vi "Experiment_1b.vi"() -> ()   [LabVIEW 2019]
uses:
  <vilib>/measure/NI_MABase.lvlib
panel:
  out "Modulating Filtered Signal":dynamicdata(graph)
  in  "sampling info":cluster{"Fs":dbl, "#s":dbl}={"Fs"=1000.0, "#s"=1000.0} {"Fs" format="%.2p"}
  in  "phase":dbl format="%.2p"
  out "Demodulated Signal":dynamicdata(graph)=[{"t0"=timestamp(0 s since 1904-01-01), "dt"=0.0001, "Y"=array[1000 elements], "attributes"=variant("NI_ChannelName"=variant(string "Filtered"))}]
  out "Modulated Signal":dynamicdata(graph)
  out "Carrier Signal":waveform(dbl)(graph)={"t0"=timestamp(0 s since 1904-01-01), "dt"=0.0001, "Y"=array[1000 elements]}
  out "Modulating Unfiltered Signal":waveform(dbl)(graph)={"t0"=timestamp(0 s since 1904-01-01), "dt"=0.0001, "Y"=array[1000 elements]}
  in  "amplitude 2":dbl=1.0 format="%0.2p"
  in  "frequency 2":dbl=1000.0 format="%0.2p"
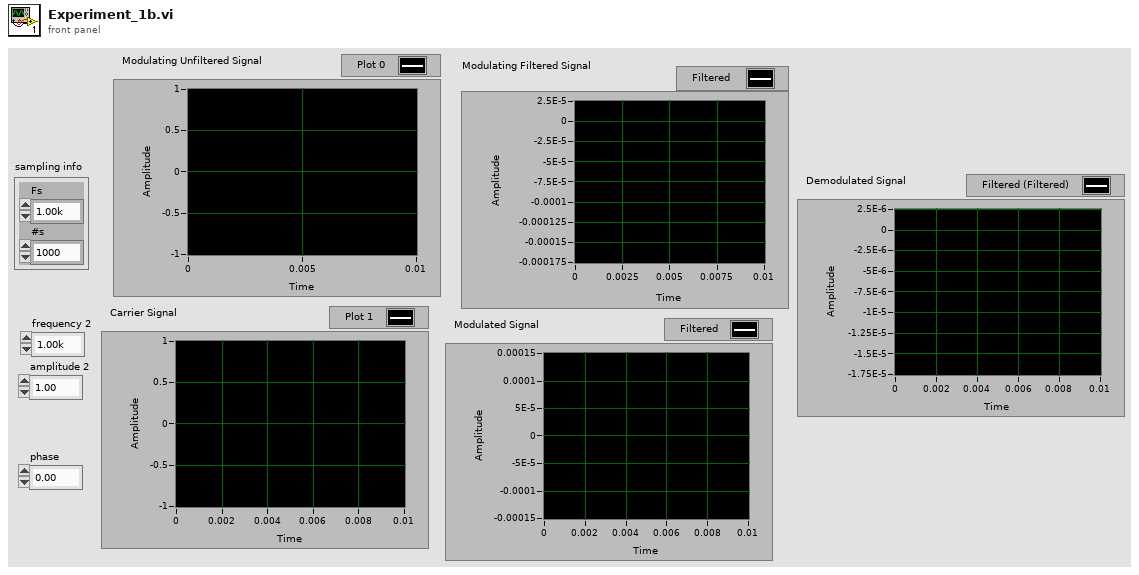
[diagram p1: front panel]
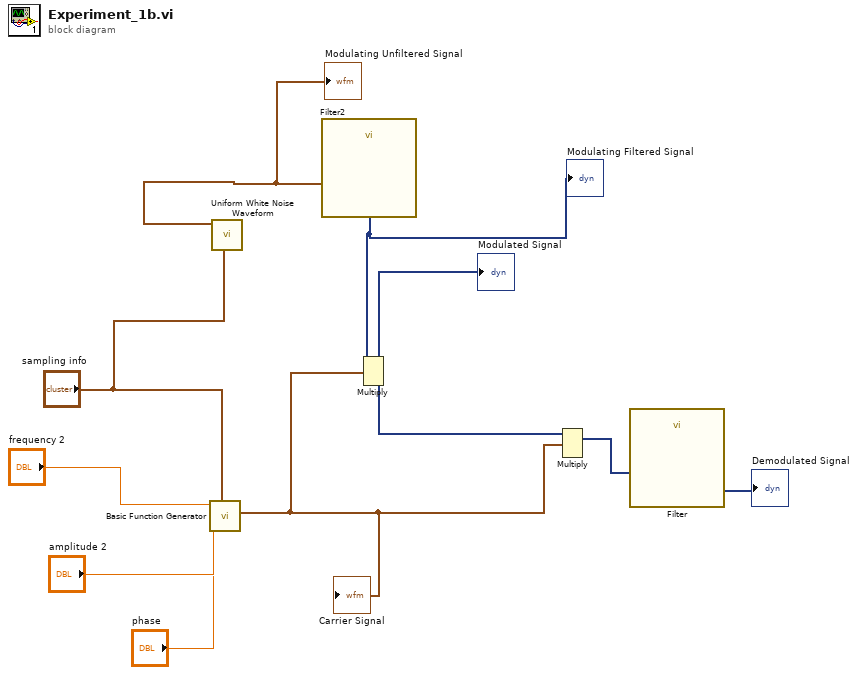
[diagram p0: block diagram]
diagram:
  n1 = call <vilib>:"Basic Function Generator.vi"("sampling info"="sampling info", "phase"="phase", "amplitude"="amplitude 2", "frequency"="frequency 2") -> ("signal out"=w7:waveform(dbl))  [unwired: 5 in, 2 out]
  "Carrier Signal" <- w7
  n2 = call <vilib>:"Uniform White Noise Waveform.vi"("sampling info"="sampling info") -> ("signal out"=w3:waveform(dbl))  [unwired: 9 in, 1 out]
  "Modulating Unfiltered Signal" <- w3
  n3 = call "Filter2"("Signal"=w3) -> ("Filtered Signal"=w2:dynamicdata)  [unwired: 9 in, 1 out]
  "Modulating Filtered Signal" <- w2
  n4 = Multiply(1:w7, 2:w2) -> (0:w8:dynamicdata)  [unwired: 1 in, 1 out]
  "Modulated Signal" <- w8
  n5 = Multiply(1:w7, 2:w8) -> (0:w6:dynamicdata)  [unwired: 1 in, 1 out]
  n6 = call "Filter"("Signal"=w6) -> ("Filtered Signal"=→"Demodulated Signal":dynamicdata)  [unwired: 9 in, 1 out]
